vi "CPD Topo & GridSpectr.vi"(6 "Internal use":string, 7 "Grid param":T1 {"height (m)" format="%#_6p"; "width (m)" format="%#_6p"; "center Y (m)" format="%#_6p"; "center X (m)" format="%#_6p"}, 8 "Error in (no error)":errorcluster, 9 "Points Y/Index Y":i32, 10 "Points X/Index X":i32, 11 "Method":enum16{"init", "run", "end"}(ring)) -> (0 "Error out":errorcluster)   [LabVIEW 2017]
doc: "Example of a measurement VI to be used in the \"Experiments on a Grid\" tool as external VI.\n\nThis example measure the topography and spectroscopy data. The spectroscopy measurements are taken on a subgrid. The data are saved to a sxm and a binary file.\n\n- Nanonis Programming Interface -"
uses:
  Instance           1 53Saved   Grid Measurements Example - Topo & GridSpectr .vi
  <userlib>/Nanonis Prog Interface V5/Nanonis Prog Interface.lvlib
panel:
  in  "Y subgrid spacing":u16=4
  in  "X subgrid spacing":u16=4
  # "Example of a measurement VI to be used in the \"Experiments on a Grid\" tool as external VI.\n\nThis example measure the topography and spectroscopy data. The spectroscopy measurements are taken on a subgrid. The data are saved to a sxm and a binary file.\n\nTo use it, set up the bias spectroscopy module to record the desired channels and set all other spectroscopy parameters. Then, set up the experiments on a grid module to use this VI as \"external VI\". On this VI's front panel, adjust the subgrid spacing.\n\n\"Experiments on a Grid\" will first (before starting the measurements) call the external VI with the \"init\" method, passing the grid resolution (Points X, Points Y) and the grid dimensions (Grid).\nThen, for the measurements, the external VI will be called with the \"run\" method, passing the current X and Y indices (Index X, Index Y).\nAfter the last measurement, the external VI will be called using the \"end\" method.\n\nSee diagram for more information about this example."
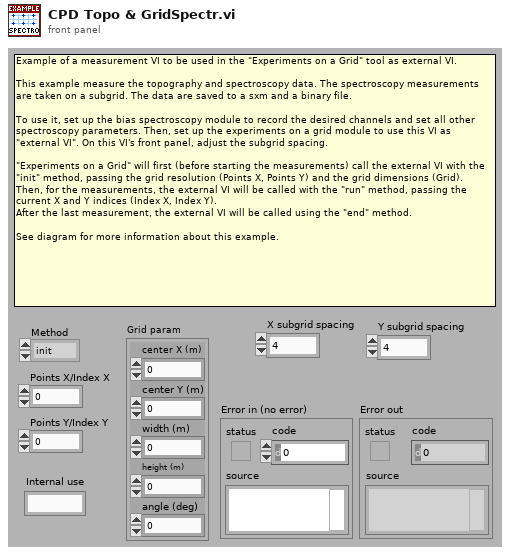
[diagram p1: front panel]
types:
  T1 = cluster{"center X (m)":sgl, "center Y (m)":sgl, "width (m)":sgl, "height (m)":sgl, "angle (deg)":sgl}
  T2 = cluster{"center X":sgl, "center Y":sgl, "angle":sgl, "width":sgl, "height":sgl, "# pixels":i32, "# lines":i32}
  T3 = cluster{"Name":string, "Calibration":sgl, "Offset":sgl, "Channel index":i32}[]
  T4 = cluster{"up/down":bool, "time/line":sgl, "start time":timestamp, "end time":timestamp}
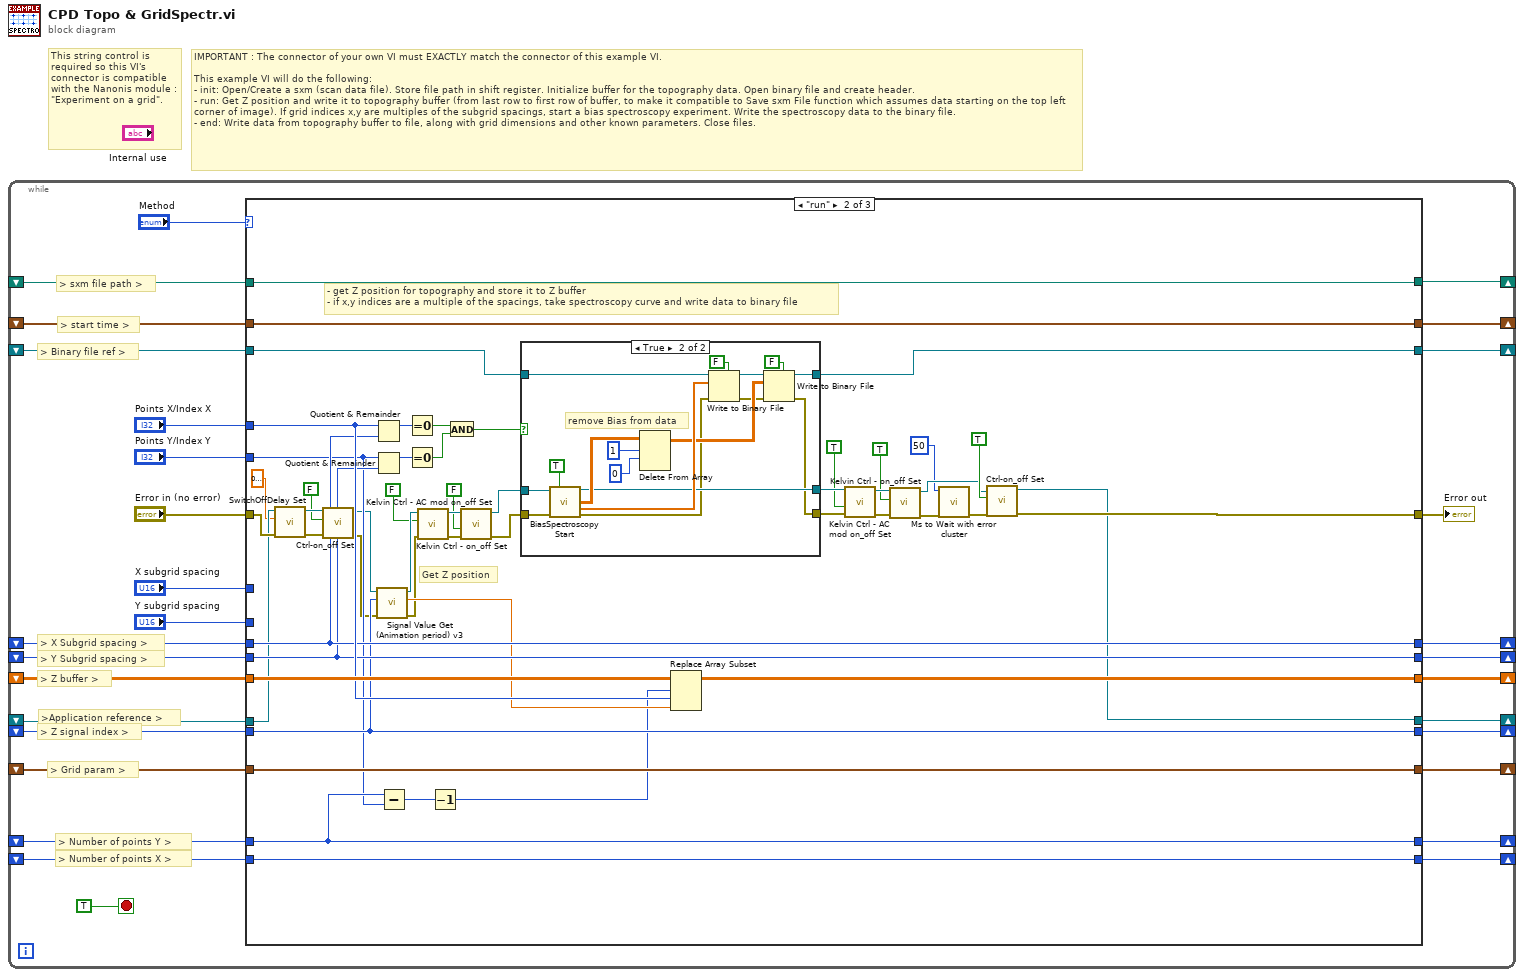
[diagram p0: block diagram]
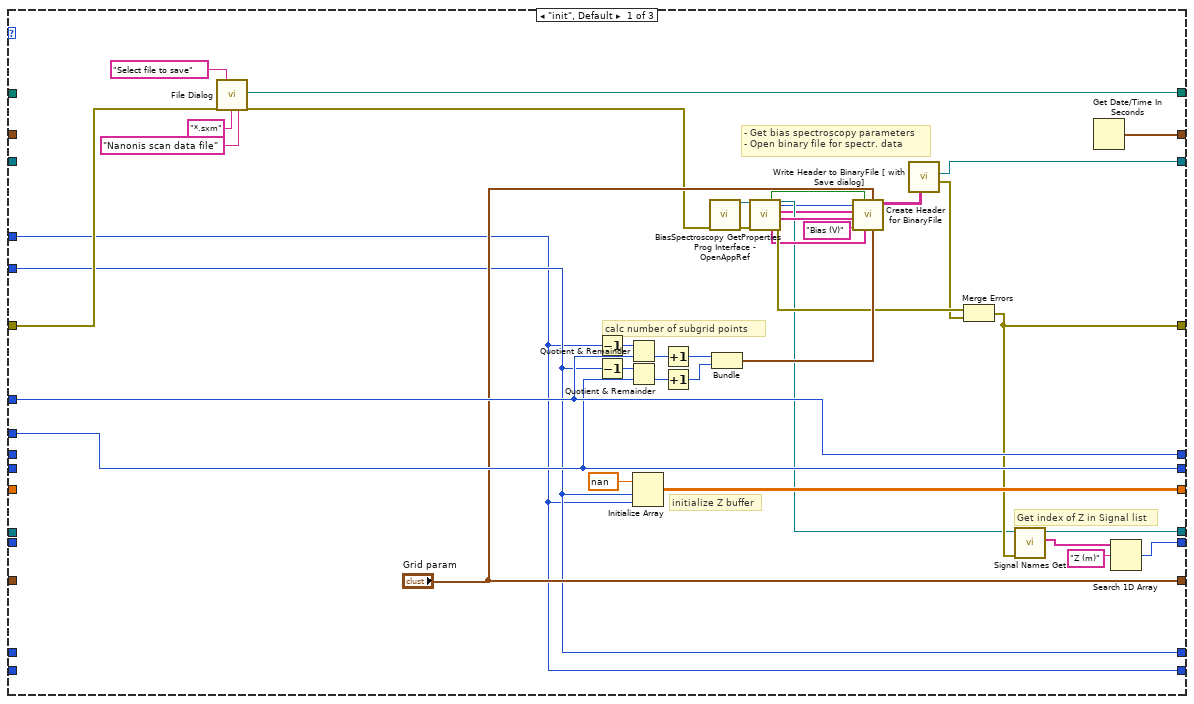
[diagram p2: hidden frame]
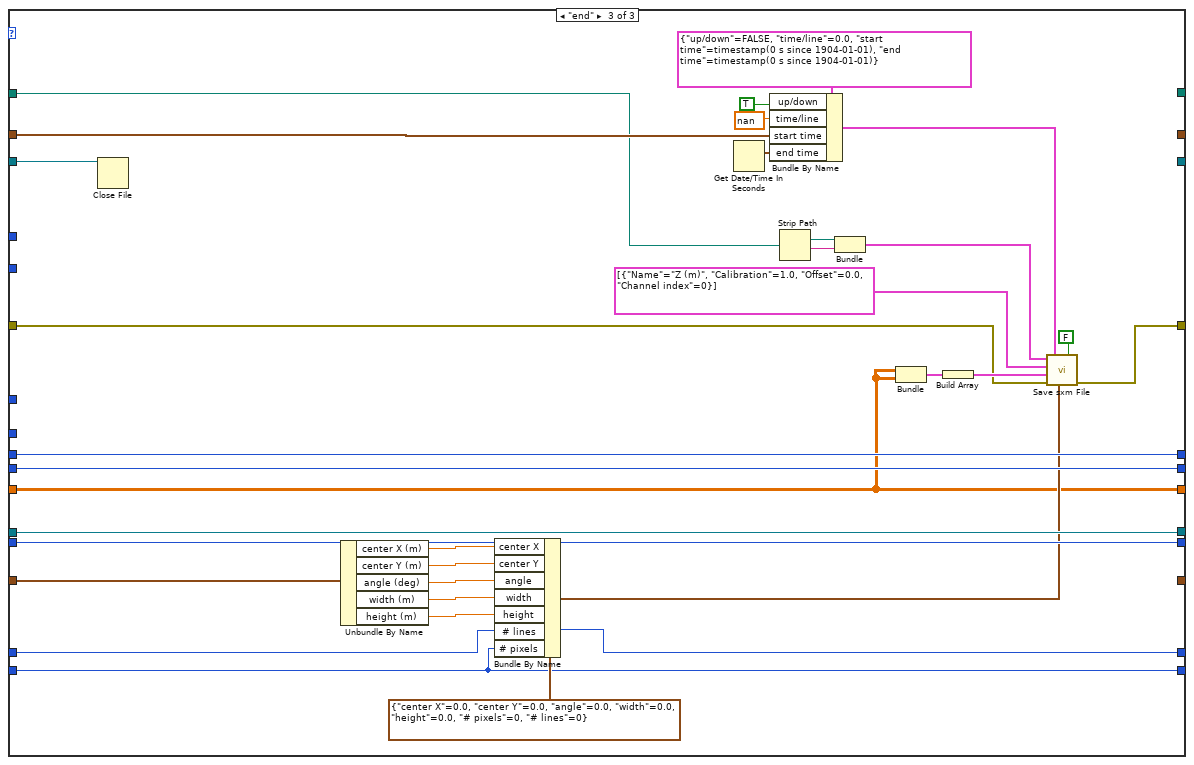
[diagram p4: hidden frame]
diagram:
  # "This string control is required so this VI's connector is compatible with the Nanonis module : \"Experiment on a grid\"."
  # "IMPORTANT : The connector of your own VI must EXACTLY match the connector of this example VI.\n\nThis example VI will do the following:\n- init: Open/Create a sxm (scan data file). Store file path in shift register. Initialize buffer for the topography data. Open binary file and create header.\n- run: Get Z position and write it to topography buffer (from last row to first row of buffer, to make it compatible to Save sxm File function which assumes data starting on the top left corner of image). If grid indices x,y are multiples of the subgrid spacings, start a bias spectroscopy experiment. Write the spectroscopy data to the binary file.\n- end: Write data from topography buffer to file, along with grid dimensions and other known parameters. Close files."
  n1 = while {
    shift-right: [w5] -> _
    shift-left: _ -> [w28]
    shift-right: [w23] -> _
    shift-left: _ -> [w22]
    shift-right: [w20] -> _
    shift-left: _ -> [w21]
    shift-right: [w19] -> _
    shift-left: _ -> [w18]
    shift-right: [w12] -> _
    shift-left: _ -> [w14]
    shift-right: [w13] -> _
    shift-left: _ -> [w15]
    shift-right: [w11] -> _
    shift-left: _ -> [w10]
    shift-right: [w9] -> _
    shift-left: _ -> [w8]
    shift-right: [w7] -> _
    shift-left: _ -> [w6]
    shift-right: [w4] -> _
    shift-left: _ -> [w3]
    shift-right: [w2] -> _
    shift-left: _ -> [w1]
    stop <- TRUE stop-if-true
    # "> Number of points X >"
    # "> Number of points Y >"
    # "> Grid param >"
    # "> start time >"
    # ">Application reference >"
    # "> Y Subgrid spacing >"
    # "> X Subgrid spacing >"
    # "> Z signal index >"
    # "> Binary file ref >"
    # "> Z buffer >"
    # "> sxm file path >"
    n2 = case shown="\"run\"" "Method" {
      tunnel: [w35 w120 _] -> w5
      tunnel: w28 -> [_ w120 w161]
      tunnel: "Error in (no error)" -> [w37 w98 w153]
      tunnel: [w47 w86 w152] -> w26
      tunnel: "Points X/Index X" -> [w31 w115 _]
      tunnel: "Points Y/Index Y" -> [w32 w101 _]
      tunnel: [w69 w118 w141] -> w23
      tunnel: w22 -> [_ w119 w141]
      tunnel: w21 -> [_ w117 w171]
      tunnel: [w60 w116 _] -> w20
      tunnel: [w58 w107 w172] -> w19
      tunnel: w18 -> [_ w107 w172]
      tunnel: "X subgrid spacing" -> [w57 _ _]
      tunnel: "Y subgrid spacing" -> [w56 _ _]
      tunnel: w15 -> [_ w109 w170]
      tunnel: w14 -> [_ w108 w169]
      tunnel: [w57 w109 w170] -> w13
      tunnel: [w56 w108 w169] -> w12
      tunnel: [w43 w85 w168] -> w11
      tunnel: w10 -> [_ w95 w168]
      tunnel: ["Grid param" w104 _] -> w9
      tunnel: w8 -> [_ w104 w151]
      tunnel: [w39 w105 _] -> w7
      tunnel: w6 -> [_ w105 w162]
      tunnel: [w32 w102 w142] -> w4
      tunnel: w3 -> [_ w102 w142]
      tunnel: [w31 w103 w143] -> w2
      tunnel: w1 -> [_ w103 w143]
      frame "init", Default {
        # "- Get bias spectroscopy parameters\n- Open binary file for spectr. data"
        # "initialize Z buffer"
        # "calc number of subgrid points"
        # "Get index of Z in Signal list"
        n3 = call "File Dialog"("prompt"="Select file to save", "error in"=w37, "pattern (all files)"="*.sxm" ("pattern"), "pattern label"="Nanonis scan data file") -> ("selected path"=w35:path, "error out"=w36:errorcluster)  [unwired: 8 in, 2 out]
        n4 = Decrement(x=w31) -> (x-1=w55:i32)
        n5 = Decrement(x=w32) -> (x-1=w54:i32)
        n6 = Quotient & Remainder(x=w55, y=w57) -> (floor(x/y)=w53:i32)  [unwired: 1 out]
        n7 = Quotient & Remainder(x=w54, y=w56) -> (floor(x/y)=w52:i32)  [unwired: 1 out]
        n8 = Initialize Array(sgl nan ("element"), w32, w31) -> (w69:sgl[][])
        n9 = Increment(x=w53) -> (x+1=w51:i32)
        n10 = Increment(x=w52) -> (x+1=w50:i32)
        n11 = call <userlib>:"Prog Interface - OpenAppRef.vi"("Error in (no error)"=w36) -> ("Error out"=w48:errorcluster, "Application reference"=w46:refnum<vi>)  [unwired: 5 in]
        n12 = Bundle(w51, w50) -> (w64:cluster{i32, i32})  [unwired: 1 in]
        n13 = call <userlib>:"BiasSpectroscopy GetProperties.vi"("Application ref in"=w46, "Error in (no error)"=w48) -> ("Backward sweep"=w65:bool, "Application ref out"=w45:refnum<vi>, "Number of points"=w42:i32, "Channels"=w41:string[], "Parameters"=w63:string[], "Fixed parameters"=w49:string[], "Error out"=w62:errorcluster)  [unwired: 6 in, 1 out]
        n14 = call <userlib>:"Create Header for BinaryFile.vi"("Grid points"=w64, "Grid param"="Grid param", "Fixed parameters"=w49, "Backward sweep"=w65, "Sweep signal"="Bias (V)" ("Sweep Signal"), "Parameters"=w63, "Channels"=w41, "Points per sweep"=w42) -> ("Header (fixed attributes)"=w67:string[][])  [unwired: 3 in]
        n15 = call <userlib>:"Write Header to BinaryFile [ with Save dialog].vi"("Fixed Attributes"=w67) -> ("Error out"=w61:errorcluster, "File ref"=w60:refnum<file>)  [unwired: 7 in, 2 out]
        n16 = Merge Errors(w62, w61) -> (w47:errorcluster)
        n17 = call <userlib>:"Signal Names Get.vi"("error in (no error)"=w47, "Application ref in"=w45) -> ("Signals Names"=w44:string[], "Application ref out"=w43:refnum<vi>)  [unwired: 5 in, 1 out]
        n18 = Get Date/Time In Seconds() -> (seconds since 1Jan1904=w39:timestamp)
        n19 = Search 1D Array(1D array=w44, element="Z (m)") -> (index of element=w58:i32)  [unwired: 1 in]
      }
      frame "run" {
        # "Get Z position"
        # "- get Z position for topography and store it to Z buffer\n- if x,y indices are a multiple of the spacings, take spectroscopy curve and write data to binary file"
        n20 = call <userlib>:"SwitchOffDelay Set.vi"("error in (no error)"=w98, "Switch off Delay (s)"=0.9999999999999999, "Application ref in"=w95) -> ("error out"=w97:errorcluster, "Application ref out"=w96:refnum<vi>)  [unwired: 7 in]
        n21 = call <userlib>:"Ctrl-on_off Set.vi"("error in (no error)"=w97, "Z Controller ON/OFF"=FALSE, "Application ref in"=w96) -> ("error out"=w92:errorcluster, "Application ref out"=w91:refnum<vi>)  [unwired: 7 in]
        n22 = Quotient & Remainder(x=w115, y=w109) -> (x-y*floor(x/y)=w114:i32)  [unwired: 1 out]
        n23 = Quotient & Remainder(x=w101, y=w108) -> (x-y*floor(x/y)=w113:i32)  [unwired: 1 out]
        n24 = call <userlib>:"Signal Value Get (Animation period) v3.vi"("error in (no error)"=w92, "Signal index (0-127)"=w107, "Application ref in"=w91) -> ("error out"=w87:errorcluster, "Signal value"=w106:sgl, "Application ref out"=w90:refnum<vi>)  [unwired: 5 in]
        n25 = Subtract(x=w102, y=w101) -> (x-y=w100:i32)
        n26 = Equal To 0?(x=w114) -> (x = 0?=w112:bool)
        n27 = Equal To 0?(x=w113) -> (x = 0?=w111:bool)
        n28 = call <userlib>:"Kelvin Ctrl - on_off Set.vi"("error in (no error)"=w87, "Kelvin controller ON/OFF"=FALSE, "Application ref in"=w90) -> ("error out"=w93:errorcluster, "Application ref out"=w94:refnum<vi>)  [unwired: 7 in]
        n29 = Decrement(x=w100) -> (x-1=w99:i32)
        n30 = And(x=w112, y=w111) -> (x .and. y?=w110:bool)
        n31 = call <userlib>:"Kelvin Ctrl - AC mod on_off Set.vi"("error in (no error)"=w93, "Modulation ON/OFF"=FALSE, "Application ref in"=w94) -> ("error out"=w88:errorcluster, "Application ref out"=w89:refnum<vi>)  [unwired: 7 in]
        n32 = case shown="True" w110 {
          tunnel: [w122 w124] -> w78
          tunnel: w117 -> [w123 w140]
          tunnel: [w123 w138] -> w116
          tunnel: w88 -> [w122 w137]
          tunnel: w89 -> [w121 w129]
          tunnel: [w121 w128] -> w79
          frame False {
            # "Point indices aren't multiple of subgrid spacing\n=> no spectroscopy at this point"
          }
          frame True {
            # "remove Bias from data"
            n33 = call <userlib>:"BiasSpectroscopy Start.vi"("Application ref in"=w129, "Get data (F)"=TRUE ("Get Data (F)"), "Error in (no error)"=w137) -> ("Application ref out"=w128:refnum<vi>, "Data"=w136:sgl[][], "Parameters"=w135:sgl[], "Error out"=w126:errorcluster)  [unwired: 8 in, 1 out]
            n34 = Delete From Array(array=w136, length=1, index (row)=0 ("index")) -> (array with subset deleted=w134:sgl[][])  [unwired: 1 in, 1 out]
            n35 = Write to Binary File(file (use dialog)=w140, data=w135, error in=w126, 5:FALSE ("prepend array or string size? (T)")) -> (refnum out=w139:refnum<file>, error out=w125:errorcluster)  [unwired: 2 in, 1 out]
            n36 = Write to Binary File(file (use dialog)=w139, data=w134, error in=w125, 5:FALSE ("prepend array or string size? (T)")) -> (refnum out=w138:refnum<file>, error out=w124:errorcluster)  [unwired: 2 in, 1 out]
          }
        }
        n37 = Replace Array Subset(array=w119, new element=w106, index (row)=w99, index (col)=w115) -> (w118:sgl[][])
        n38 = call <userlib>:"Kelvin Ctrl - AC mod on_off Set.vi"("error in (no error)"=w78, "Modulation ON/OFF"=TRUE, "Application ref in"=w79) -> ("error out"=w76:errorcluster, "Application ref out"=w77:refnum<vi>)  [unwired: 7 in]
        n39 = call <userlib>:"Kelvin Ctrl - on_off Set.vi"("error in (no error)"=w76, "Kelvin controller ON/OFF"=TRUE, "Application ref in"=w77) -> ("error out"=w72:errorcluster, "Application ref out"=w73:refnum<vi>)  [unwired: 7 in]
        n40 = call <userlib>:"Ms to Wait with error cluster.vi"("error in (no error)"=w72, "milliseconds to wait"=50) -> ("error out"=w71:errorcluster)  [unwired: 4 in, 1 out]
        n41 = call <userlib>:"Ctrl-on_off Set.vi"("error in (no error)"=w71, "Z Controller ON/OFF"=TRUE, "Application ref in"=w73) -> ("error out"=w86:errorcluster, "Application ref out"=w85:refnum<vi>)  [unwired: 7 in]
      }
      frame "end" {
        n42 = Close File(refnum=w171) -> ()  [unwired: 1 in, 2 out]
        n43 = Unbundle By Name(w151) -> ("center X (m)"=w149:sgl, "center Y (m)"=w148:sgl, "angle (deg)"=w147:sgl, "width (m)"=w146:sgl, "height (m)"=w145:sgl)
        n44 = Bundle By Name(cluster=T2 {"center X"=0.0, "center Y"=0.0, "angle"=0.0, "width"=0.0, "height"=0.0, "# pixels"=0, "# lines"=0} ("Scanfield"), "center X"=w149, "center Y"=w148, "angle"=w147, "width"=w146, "height"=w145, "# lines"=w142, "# pixels"=w143) -> (w144:T2)
        n45 = Get Date/Time In Seconds() -> (seconds since 1Jan1904=w159:timestamp)
        n46 = Bundle By Name(cluster=T4 {"up/down"=FALSE, "time/line"=0.0, "start time"=timestamp(0 s since 1904-01-01), "end time"=timestamp(0 s since 1904-01-01)} ("Scan param"), "up/down"=TRUE, "time/line"=sgl nan ("input 7"), "start time"=w162, "end time"=w159) -> (w160:T4)
        n47 = Strip Path(path=w161) -> (stripped path=w156:path, name=w155:string)
        n48 = Bundle("stripped path"=w156, "name"=w155) -> (w154:cluster{"stripped path":path, "name":string})  [unwired: 1 in]
        n49 = Bundle(w141, w141) -> (w167:cluster{sgl[][], sgl[][]})  [unwired: 1 in]
        n50 = Build Array(w167) -> (w166:cluster{sgl[][], sgl[][]}[])
        n51 = call <userlib>:"Save sxm File.vi"("Auto file naming? (T)"=FALSE, "Scanfield"=w144, "Scan param"=w160, "error in (no error)"=w153, "Channels data"=w166, "Channels config"=T3 [{"Name"="Z (m)", "Calibration"=1.0, "Offset"=0.0, "Channel index"=0}], "Filename control"=w154) -> ("error out"=w152:errorcluster)  [unwired: 2 in, 2 out]
      }
    }
    "Error out" <- w26
  }
